vi "ATS get force.vi"(11 "索引":i32=7) -> (3 "数值":i32)   [LabVIEW 2018]
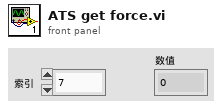
[diagram p1: front panel]
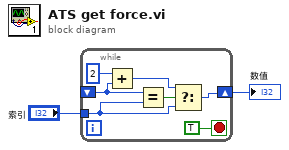
[diagram p0: block diagram]
diagram:
  n1 = while {
    shift-right: [w7] -> w2
    shift-left: _ -> [w5]
    tunnel: "索引" -> [w4]
    stop <- TRUE stop-if-true
    n2 = Add(x=2, y=w5) -> (x+y=w8:i32)
    n3 = Equal?(x=w5, y=w4) -> (x = y?=w9:bool)
    n4 = Select(t=w8, s=w9, f=w4) -> (s? t:f=w7:i32)
  }
  "数值" <- w2
